vi "MICSD Serial Write.vi"(8 "error in (no error)":errorcluster, 10 "Write Data":T1, 11 "VISA Resource Name":refnum<visa-resource-name>) -> (0 "error out":errorcluster, 3 "DUP Visa Resource Name":refnum<visa-resource-name>)   [LabVIEW 2020]
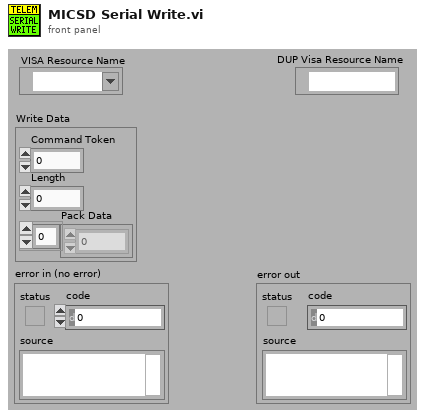
[diagram p1: front panel]
types:
  T1 = cluster{"Command Token":u8, "Length":u16, "Pack Data":u8[]}
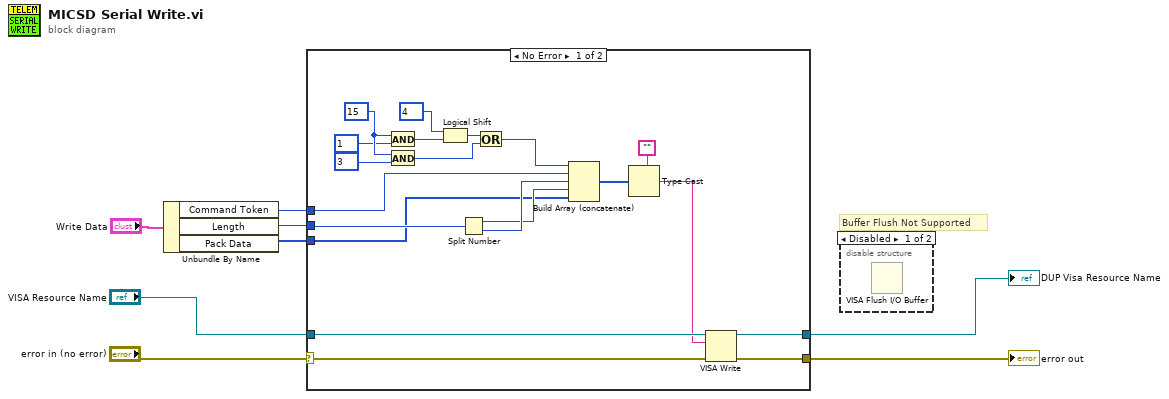
[diagram p0: block diagram]
diagram:
  # "Buffer Flush Not Supported"
  n1 = Unbundle By Name("Write Data") -> ("Command Token"=w7:u8, "Length"=w6:u16, "Pack Data"=w5:u8[])
  n2 = case shown="No Error" "error in (no error)" {
    selector: "error in (no error)" -> [w18 w29]
    tunnel: "VISA Resource Name" -> [w19 w30]
    tunnel: [w10 w30] -> w4
    tunnel: [w9 w29] -> w3
    tunnel: w7 -> [w15 _]
    tunnel: w6 -> [w14 _]
    tunnel: w5 -> [w13 _]
    frame No Error {
      w28 = u8 15 ("Source")
      n3 = And(x=w28, y=u8 1 ("Source")) -> (x .and. y?=w27:u8)
      n4 = And(x=w28, y=u8 3 ("Source")) -> (x .and. y?=w25:u8)
      n5 = Logical Shift(y=u8 4 ("Source"), x=w27) -> (x << y=w26:u8)
      n6 = Split Number(x=w14) -> (hi(x)=w22:u8, lo(x)=w23:u8)
      n7 = Or(x=w26, y=w25) -> (x .or. y?=w24:u8)
      n8 = Build Array (concatenate)(w24, w15, w23, w22, w13) -> (w21:u8[])
      n9 = Type Cast(type="", x=w21) -> (*(type *) &x=w11:string)
      n10 = VISA Write(VISA resource name=w19, write buffer=w11, error in (no error)=w18) -> (VISA resource name out=w10:refnum<visa-resource-name>, error out=w9:errorcluster)  [unwired: 1 out]
    }
    frame Error {
    }
  }
  "DUP Visa Resource Name" <- w4
  "error out" <- w3
  n11 = disable-structure shown="Disabled" {
    frame Disabled {
      n12 = VISA Flush I/O Buffer() -> ()  [unwired: 3 in, 2 out]
    }
    frame Enabled {
    }
  }
